vi "Create Pattern Script(DataCompare).vi"(7 "Num of wait cycle for read":i8, 8 "error in (no error)":errorcluster, 11 "Data":u8[](array[numeric])) -> (0 "error out":errorcluster, 3 "String":string)   [LabVIEW 2018, in "BML_Frame_Root.lvclass"]
uses:
  BML_Frame_Root.lvclass
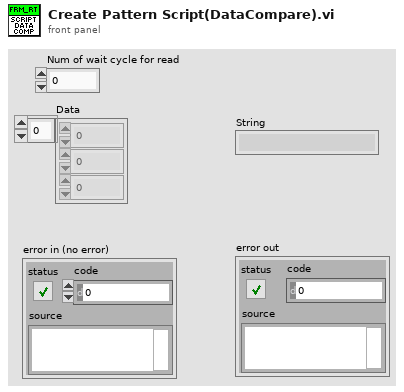
[diagram p1: front panel]
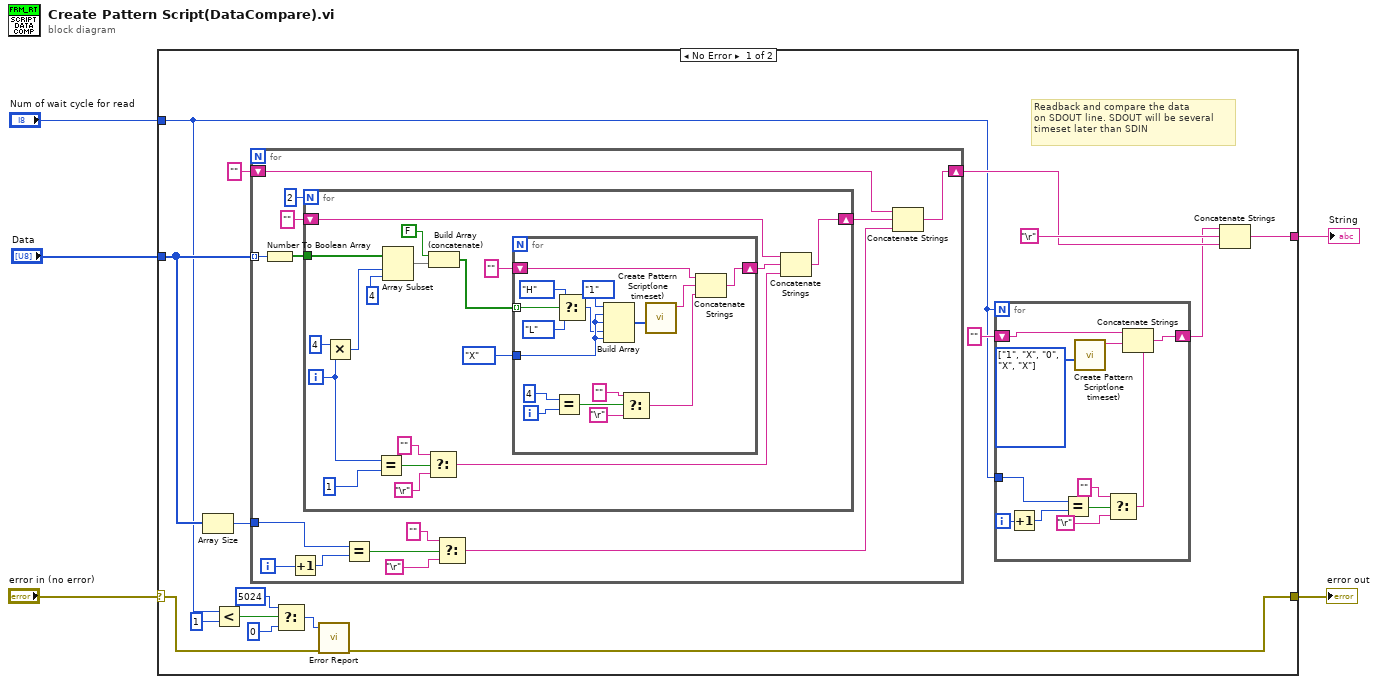
[diagram p0: block diagram]
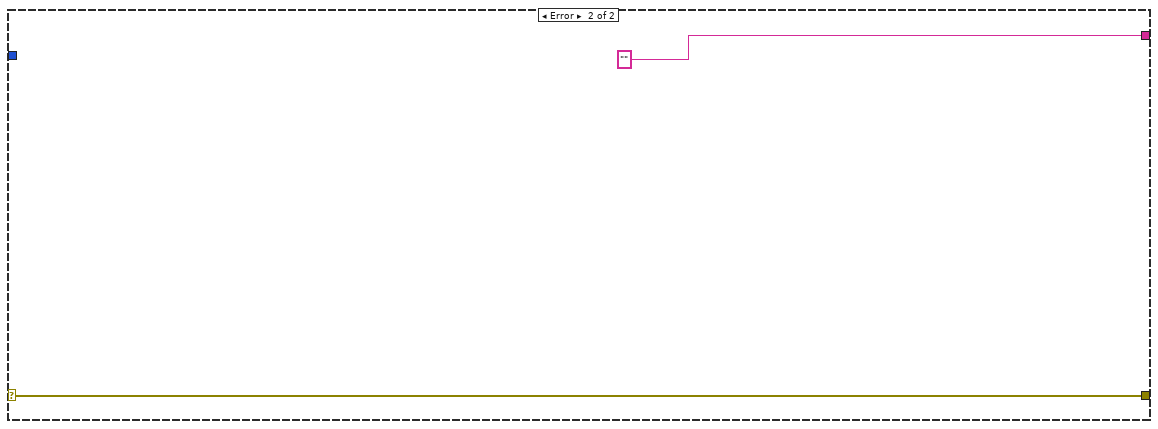
[diagram p2: hidden frame]
diagram:
  n1 = case shown="No Error" "error in (no error)" {
    selector: "error in (no error)" -> [w7 w81]
    tunnel: [w16 ""] -> w4
    tunnel: [w6 w81] -> w3
    tunnel: "Data" -> [w21 _]
    tunnel: "Num of wait cycle for read" -> [w8 _]
    frame No Error {
      # "Readback and compare the data\non SDOUT line. SDOUT will be several \ntimeset later than SDIN"
      n2 = Array Size(array=w21) -> (size(s)=w20:i32)
      n3 = Less?(x=w8, y=i8 1) -> (x < y?=w10:bool)
      n4 = for {
        tunnel: w21 -> [w43] mode=indexing
        tunnel: w20 -> [w40]
        shift-right: [w34] -> w17
        shift-left: "" -> [w33]
        i -> [w42]
        n5 = Number To Boolean Array(number=w43) -> (Boolean array=w46:bool[])
        n6 = Increment(x=w42) -> (x+1=w41:i32)
        n7 = for {
          N: 2 -> [_]
          tunnel: w46 -> [w64]
          shift-right: [w49] -> w36
          shift-left: "" -> [w48]
          i -> [w56]
          n8 = Multiply(x=4 ("y"), y=w56) -> (x*y=w62:i32)
          n9 = Equal?(x=w56, y=1) -> (x = y?=w54:bool)
          n10 = Array Subset(array=w64, index=w62, length=4) -> (w61:bool[])
          n11 = Select(t="", s=w54, f="\r") -> (s? t:f=w50:string)
          n12 = Build Array (concatenate)(FALSE, w61) -> (w58:bool[])
          n13 = for {
            tunnel: w58 -> [w80] mode=indexing
            shift-right: [w73] -> w51
            shift-left: "" -> [w72]
            tunnel: enum16{"0", "1", "L", "H", "X", "V", "D", "M"}."X" ("element") -> [w66]
            i -> [w78]
            n14 = Equal?(x=4, y=w78) -> (x = y?=w76:bool)
            n15 = Select(t=enum16{"0", "1", "L", "H", "X", "V", "D", "M"}."H" ("PinState"), s=w80, f=enum16{"0", "1", "L", "H", "X", "V", "D", "M"}."L") -> (s? t:f=w65:enum16{"0", "1", "L", "H", "X", "V", "D", "M"})
            n16 = Build Array(enum16{"0", "1", "L", "H", "X", "V", "D", "M"}."1" ("element"), w66, w66, w65, w66) -> (w70:enum16{"0", "1", "L", "H", "X", "V", "D", "M"}[])
            n17 = Select(t="", s=w76, f="\r") -> (s? t:f=w71:string)
            n18 = call "Create Pattern Script(one timeset).vi"("PinState"=w70) -> ("string out"=w69:string)  [unwired: 10 in]
            n19 = Concatenate Strings(w72, w69, w71) -> (w73:string)
          }
          n20 = Concatenate Strings(w48, w51, w50) -> (w49:string)
        }
        n21 = Equal?(x=w40, y=w41) -> (x = y?=w37:bool)
        n22 = Select(t="", s=w37, f="\r") -> (s? t:f=w35:string)
        n23 = Concatenate Strings(w33, w36, w35) -> (w34:string)
      }
      n24 = Select(t=i16 5024, s=w10, f=i16 0 ("Error Code")) -> (s? t:f=w13:i16)
      n25 = call "Error Report.vi"("error in (no error)"=w7, "Error Code"=w13) -> ("error out"=w6:errorcluster)  [unwired: 9 in]
      n26 = for {
        N: w8 -> [_]
        shift-right: [w30] -> w14
        shift-left: "" -> [w29]
        tunnel: w8 -> [w23]
        i -> [w24]
        w32 = enum16{"0", "1", "L", "H", "X", "V", "D", "M"}[] [enum."1", enum."X", enum."0", enum."X", enum."X"] items=["0", "1", "L", "H", "X", "V", "D", "M"] ("PinState")
        n27 = Increment(x=w24) -> (x+1=w28:i32)
        n28 = Equal?(x=w23, y=w28) -> (x = y?=w25:bool)
        n29 = call "Create Pattern Script(one timeset).vi"("PinState"=w32) -> ("string out"=w31:string)  [unwired: 10 in]
        n30 = Select(t="", s=w25, f="\r") -> (s? t:f=w22:string)
        n31 = Concatenate Strings(w29, w31, w22) -> (w30:string)
      }
      n32 = Concatenate Strings(w14, "\r", w17) -> (w16:string)
    }
    frame Error {
    }
  }
  "String" <- w4
  "error out" <- w3
